vi "MB Registers Manager Read.vi"(5 "Data Reference":T1, 7 "Table":T2(ring), 8 "error in (no error)":errorcluster, 10 "Length":u16, 11 "Start Address":u16) -> (0 "error out":errorcluster, 1 "Words out":u16[](array[numeric]), 4 "Bits out":bool[](array[boolean]))   [LabVIEW 2019, in "NI_modbus_upd.lvlib"]
uses:
  NI_modbus_upd.lvlib
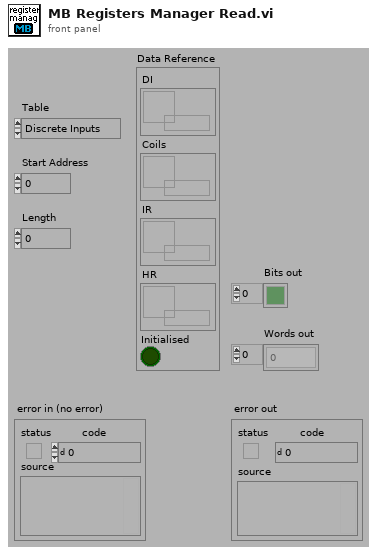
[diagram p1: front panel]
types:
  T1 = cluster{"DI":refnum<data-value>, "Coils":refnum<data-value>, "IR":refnum<data-value>, "HR":refnum<data-value>, "Initialised":bool}
  T2 = enum16{"Discrete Inputs", "Coils", "Input Registers", "Holding Registers"}
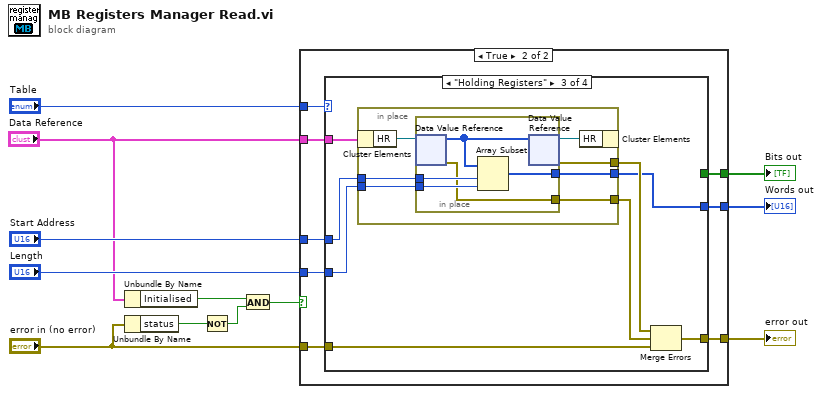
[diagram p0: block diagram]
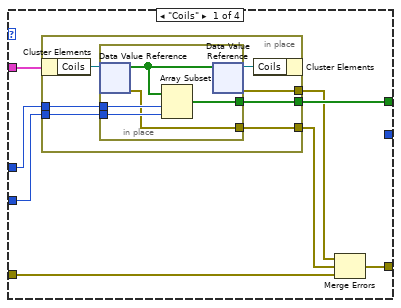
[diagram p3: hidden frame]
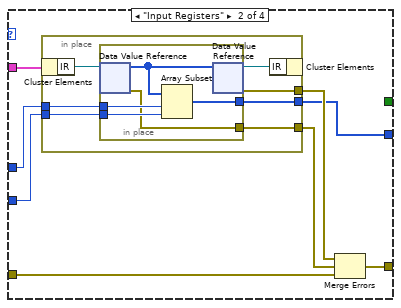
[diagram p4: hidden frame]
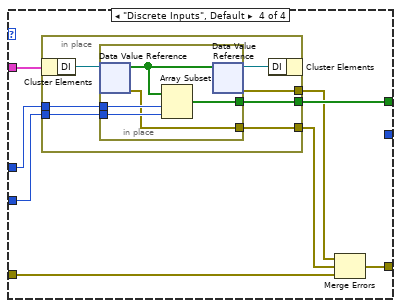
[diagram p5: hidden frame]
diagram:
  n1 = Unbundle By Name("Data Reference") -> ("Initialised"=w3:bool)
  n2 = Unbundle By Name("error in (no error)") -> ("status"=w5:bool)
  n3 = Not(x=w5) -> (.not. x?=w4:bool)
  n4 = And(x=w3, y=w4) -> (x .and. y?=w6:bool)
  n5 = case shown="True" w6 {
    tunnel: [w13 w15] -> w12
    tunnel: [_ w21] -> w11
    tunnel: [_ w20] -> w10
    tunnel: "Length" -> [_ w19]
    tunnel: "Start Address" -> [_ w18]
    tunnel: "Table" -> [_ w14]
    tunnel: "Data Reference" -> [_ w17]
    tunnel: "error in (no error)" -> [w13 w16]
    frame False {
    }
    frame True {
      n6 = case shown="\"Holding Registers\"" w14 {
        tunnel: [w29 _ _ w89] -> w21
        tunnel: [_ w42 w62 _] -> w20
        tunnel: w19 -> [w28 w49 w69 w88]
        tunnel: w18 -> [w27 w48 w68 w87]
        tunnel: w17 -> [w22 w43 w63 w82]
        tunnel: w16 -> [w26 w47 w67 w86]
        tunnel: [w23 w44 w64 w83] -> w15
        frame "Coils" {
          n7 = in-place {
            in-place-border: [w36] -> w29
            in-place-border: w28 -> [w35]
            in-place-border: w27 -> [w34]
            in-place-border: [w33] -> w25
            in-place-border: [w32] -> w24
            n8 = in-place-cluster #1(w22) -> ("Coils"=w31:refnum<data-value>)
            n9 = in-place {
              in-place-border: w34 -> [w41]
              in-place-border: w35 -> [w40]
              in-place-border: [w38] -> w36
              in-place-border: [w37] -> w32
              n10 = in-place-dvr #2(w31) -> (w39:bool[], w37:errorcluster)
              n11 = Array Subset(array=w39, index=w41, length=w40) -> (w38:bool[])
              n12 = in-place-dvr #2(w39) -> (w30:refnum<data-value>, w33:errorcluster)
            }
            n13 = in-place-cluster #1("Coils"=w30) -> ()  [unwired: 1 out]
          }
          n14 = Merge Errors(w25, w24, w26) -> (w23:errorcluster)
        }
        frame "Input Registers" {
          n15 = in-place {
            in-place-border: [w56] -> w42
            in-place-border: w49 -> [w55]
            in-place-border: w48 -> [w54]
            in-place-border: [w53] -> w46
            in-place-border: [w52] -> w45
            n16 = in-place-cluster #3(w43) -> ("IR"=w51:refnum<data-value>)
            n17 = in-place {
              in-place-border: w54 -> [w61]
              in-place-border: w55 -> [w60]
              in-place-border: [w58] -> w56
              in-place-border: [w57] -> w52
              n18 = in-place-dvr #4(w51) -> (w59:u16[], w57:errorcluster)
              n19 = Array Subset(array=w59, index=w61, length=w60) -> (w58:u16[])
              n20 = in-place-dvr #4(w59) -> (w50:refnum<data-value>, w53:errorcluster)
            }
            n21 = in-place-cluster #3("IR"=w50) -> ()  [unwired: 1 out]
          }
          n22 = Merge Errors(w46, w45, w47) -> (w44:errorcluster)
        }
        frame "Holding Registers" {
          n23 = in-place {
            in-place-border: [w76] -> w62
            in-place-border: w69 -> [w75]
            in-place-border: w68 -> [w74]
            in-place-border: [w73] -> w66
            in-place-border: [w72] -> w65
            n24 = in-place-cluster #5(w63) -> ("HR"=w71:refnum<data-value>)
            n25 = in-place {
              in-place-border: w74 -> [w81]
              in-place-border: w75 -> [w80]
              in-place-border: [w78] -> w76
              in-place-border: [w77] -> w72
              n26 = in-place-dvr #6(w71) -> (w79:u16[], w77:errorcluster)
              n27 = Array Subset(array=w79, index=w81, length=w80) -> (w78:u16[])
              n28 = in-place-dvr #6(w79) -> (w70:refnum<data-value>, w73:errorcluster)
            }
            n29 = in-place-cluster #5("HR"=w70) -> ()  [unwired: 1 out]
          }
          n30 = Merge Errors(w66, w65, w67) -> (w64:errorcluster)
        }
        frame "Discrete Inputs", Default {
          n31 = in-place {
            in-place-border: [w96] -> w89
            in-place-border: w88 -> [w95]
            in-place-border: w87 -> [w94]
            in-place-border: [w93] -> w85
            in-place-border: [w92] -> w84
            n32 = in-place-cluster #7(w82) -> ("DI"=w91:refnum<data-value>)
            n33 = in-place {
              in-place-border: w94 -> [w101]
              in-place-border: w95 -> [w100]
              in-place-border: [w98] -> w96
              in-place-border: [w97] -> w92
              n34 = in-place-dvr #8(w91) -> (w99:bool[], w97:errorcluster)
              n35 = Array Subset(array=w99, index=w101, length=w100) -> (w98:bool[])
              n36 = in-place-dvr #8(w99) -> (w90:refnum<data-value>, w93:errorcluster)
            }
            n37 = in-place-cluster #7("DI"=w90) -> ()  [unwired: 1 out]
          }
          n38 = Merge Errors(w85, w84, w86) -> (w83:errorcluster)
        }
      }
    }
  }
  "error out" <- w12
  "Bits out" <- w11
  "Words out" <- w10
